vi "NI5112.contents.vi"   [LabVIEW 2014, in "NI5112.lvlib"]
uses:
  NI5112.lvlib
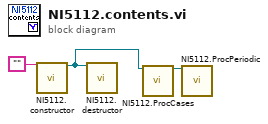
[diagram p0: block diagram]
diagram:
  n1 = call "NI5112.constructor.vi"("name"="") -> ("i ref out"=w1:refnum<vi>)  [unwired: 16 in, 2 out]
  n2 = call "NI5112.destructor.vi"("i ref in"=w1) -> ()  [unwired: 18 in, 1 out]
  n3 = call "NI5112.ProcCases.vi"("i ref in"=w1) -> ("i ref out"=w2:refnum<vi>)  [unwired: 16 in, 2 out]
  n4 = call "NI5112.ProcPeriodic.vi"("i ref in"=w2) -> ()  [unwired: 16 in, 3 out]
